vi "sub_hypotenuse.vi"(10 "x2y2":cluster{"x":dbl, "y":dbl}, 11 "x1y1":cluster{"x":dbl, "y":dbl}) -> (3 "length":dbl)   [LabVIEW 2019]
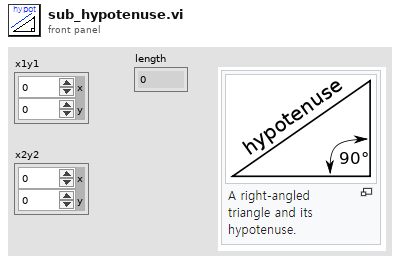
[diagram p1: front panel]
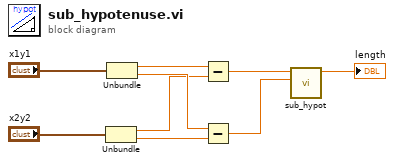
[diagram p0: block diagram]
diagram:
  n1 = Unbundle("x2y2") -> ("x"=w4:dbl, "y"=w6:dbl)
  n2 = Unbundle("x1y1") -> ("x"=w3:dbl, "y"=w5:dbl)
  n3 = Subtract(x=w3, y=w4) -> (x-y=w7:dbl)
  n4 = Subtract(x=w5, y=w6) -> (x-y=w8:dbl)
  n5 = call "sub_hypot.vi"("dy"=w8, "dx"=w7) -> ("length"=→"length":dbl)  [unwired: 9 in]
